vi "Queue Clear.vi"(8 "error in (no error)":errorcluster caption="Error In", 9 "Delete?":bool, 10 "Filter":string, 11 "Queue In":refnum<queue>) -> (0 "error out":errorcluster caption="Error Out", 3 "Queue Out":refnum<queue>)   [LabVIEW 2020]
uses:
  Queue Message.ctl
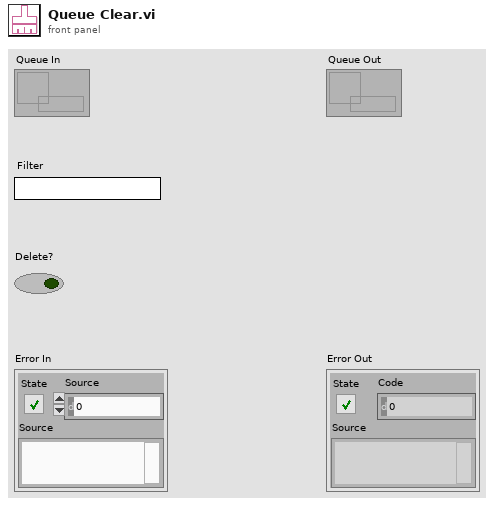
[diagram p1: front panel]
types:
  T1 = typedef "Queue Message.ctl" = cluster{"Message":string, "Data":variant}
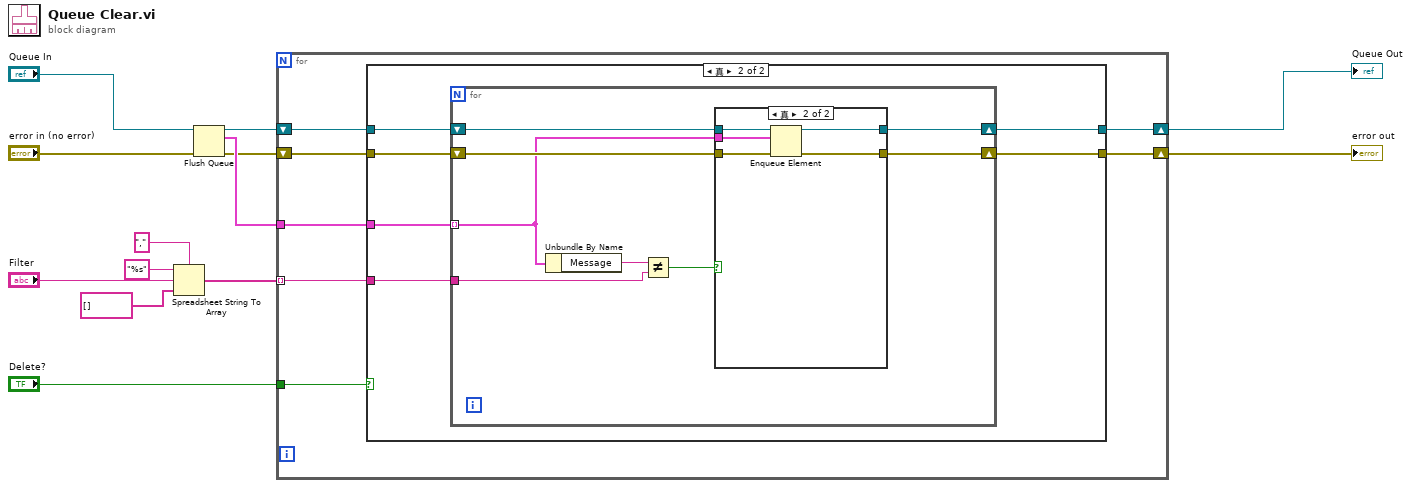
[diagram p0: block diagram]
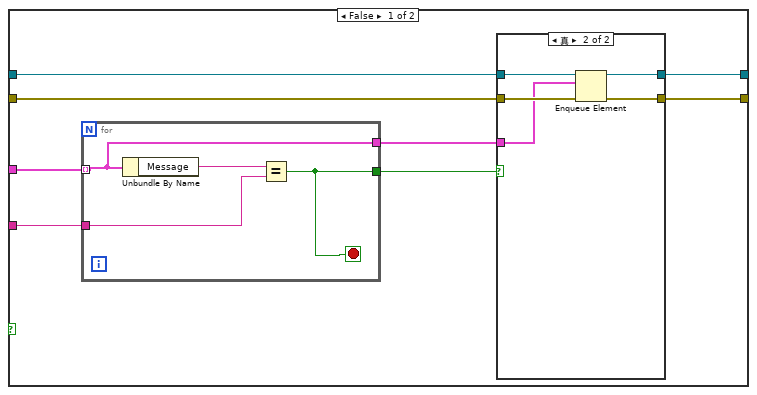
[diagram p2: hidden frame]
diagram:
  n1 = Spreadsheet String To Array(delimiter (Tab)="," ("delimiter"), format string="%s", spreadsheet string="Filter", array type (2D Dbl)=string[] []) -> (array=w11:string[])
  n2 = Flush Queue(queue="Queue In", error in (no error)="error in (no error)") -> (queue out=w3:refnum<queue>, remaining elements=w2:T1[], error out=w1:errorcluster)
  n3 = for {
    tunnel: w2 -> [w20]
    tunnel: w11 -> [w19] mode=indexing
    shift-right: [w17] -> w10
    shift-left: w3 -> [w18]
    shift-right: [w15] -> w9
    shift-left: w1 -> [w16]
    tunnel: "Delete?" -> [w14]
    n4 = case shown="真" w14 {
      tunnel: w20 -> [w28 w41]
      tunnel: w19 -> [w27 w40]
      tunnel: w18 -> [w26 w45]
      tunnel: [w25 w43] -> w17
      tunnel: w16 -> [w24 w44]
      tunnel: [w23 w42] -> w15
      frame False {
        n5 = for {
          tunnel: w28 -> [w37] mode=indexing
          tunnel: w27 -> [w38]
          tunnel: [w37] -> w22
          tunnel: [w36] -> w21
          stop <- w36 stop-if-true
          n6 = Unbundle By Name(w37) -> ("Message"=w39:string)
          n7 = Equal?(x=w39, y=w38) -> (x = y?=w36:bool)
        }
        n8 = case shown="真" w21 {
          tunnel: w26 -> [w30 w35]
          tunnel: [w30 w34] -> w25
          tunnel: w24 -> [w29 w33]
          tunnel: [w29 w32] -> w23
          tunnel: w22 -> [_ w31]
          frame False {
          }
          frame True {
            n9 = Enqueue Element(queue=w35, element=w31, error in (no error)=w33) -> (queue out=w34:refnum<queue>, error out=w32:errorcluster)  [unwired: 1 in, 1 out]
          }
        }
      }
      frame True {
        n10 = for {
          shift-right: [w52] -> w43
          shift-left: w45 -> [w53]
          shift-right: [w50] -> w42
          shift-left: w44 -> [w51]
          tunnel: w41 -> [w49] mode=indexing
          tunnel: w40 -> [w47]
          n11 = Unbundle By Name(w49) -> ("Message"=w48:string)
          n12 = Not Equal?(x=w48, y=w47) -> (x != y?=w46:bool)
          n13 = case shown="真" w46 {
            tunnel: w53 -> [w55 w60]
            tunnel: [w55 w59] -> w52
            tunnel: w51 -> [w54 w58]
            tunnel: [w54 w57] -> w50
            tunnel: w49 -> [_ w56]
            frame False {
            }
            frame True {
              n14 = Enqueue Element(queue=w60, element=w56, error in (no error)=w58) -> (queue out=w59:refnum<queue>, error out=w57:errorcluster)  [unwired: 1 in, 1 out]
            }
          }
        }
      }
    }
  }
  "Queue Out" <- w10
  "error out" <- w9
